vi "RTA4004_Oscilloscope_Fetch_2Ch_Waveform.vi"() -> ()   [LabVIEW 2017]
uses:
  <instrlib>/Rohde&Schwarz RTx Oscilloscopes/Rohde&Schwarz RTx Oscilloscopes.lvlib
panel:
  in  "Requested Record Length":i32=2000000
  out "Waveform CH2":T1(graph) caption="Waveform"
  in  "Record":bool
  in  "Description":string[](array[string])=["Measurement", "Near Football Field"]
  out "Record File Name":string
  in  "Channel 2":i32=2 caption="Channel (2)"
  out "Recorded Size":i32
  in  "Number of Loops":i32=1
  out "Current Loop":i32
  in  "Channel (1)":i32=1
  in  "Oscilloscope Resource Name":refnum<visa-resource-name>="TCPIP::192.168.10.205::INSTR" caption="VISA resource name"
  in  "Reset":bool
  in  "ID Query":bool=TRUE
  out "Waveform CH1":T1(graph) caption="Waveform"
  # "Rohde & Schwarz RTM2000 Oscilloscope Read Waveform Example"
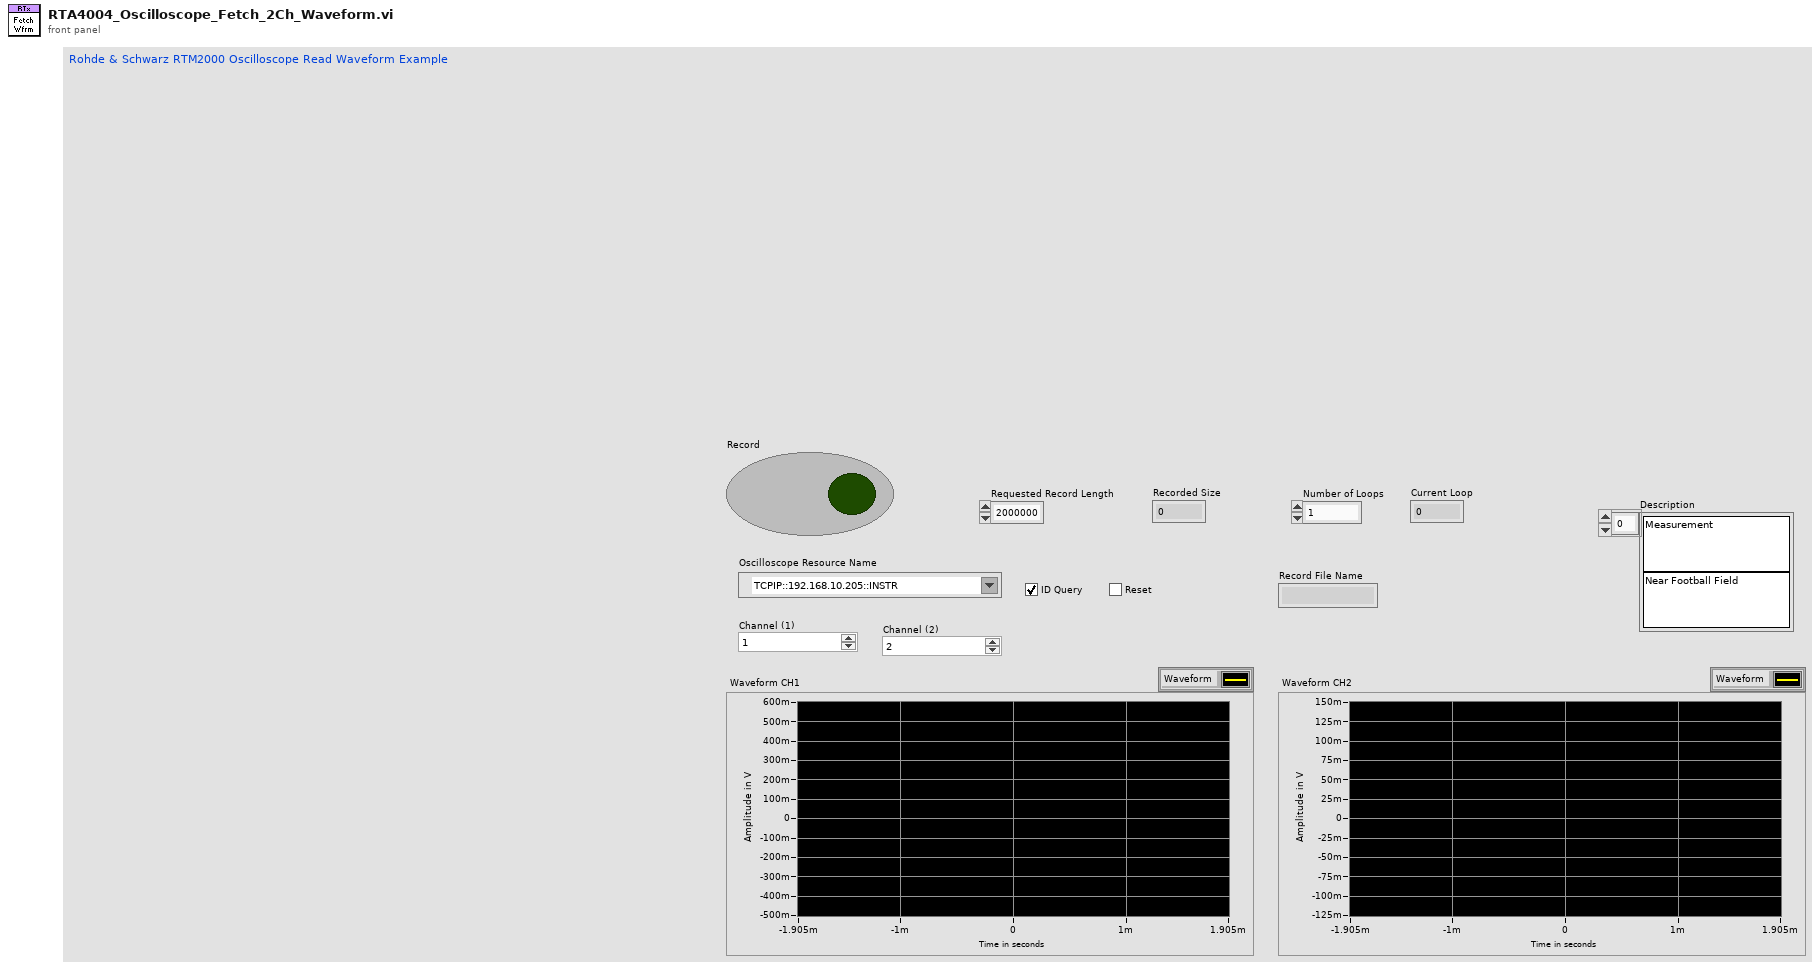
[diagram p1: front panel]
types:
  T1 = cluster{"Initial X":dbl, "X Increment":dbl, "Waveform Array":dbl[]}
  T2 = enum16{"open", "open or create", "create or replace", "create", "open (read-only)"}
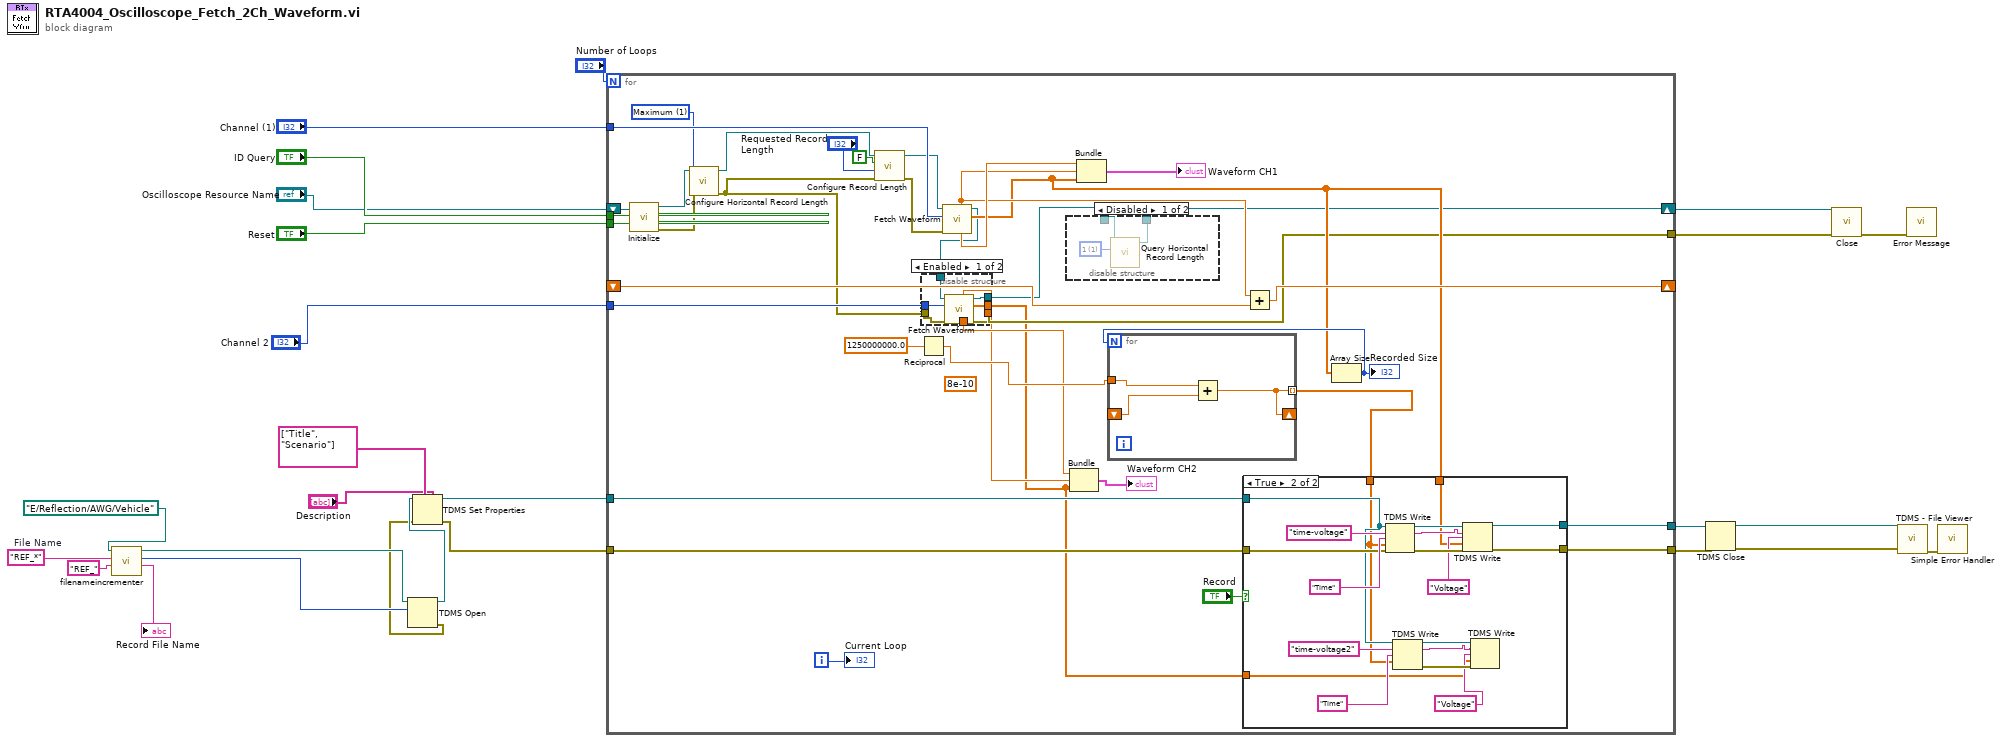
[diagram p0: block diagram]
diagram:
  w12 = "REF_*"  # File Name
  n1 = call "filenameincrementer.vi"("string"="REF_", "pattern"=w12, "Path"=path "E:/Reflection/AWG/Vehicle" ("file path")) -> ("File Name"=→"Record File Name":string, "Operation"=w8:T2, "File Path"=w7:path)  [unwired: 6 in]
  n2 = TDMS Open(10:w8, 11:w7) -> (0:w2:errorcluster, 3:w4:refnum<k34>)  [unwired: 5 in]
  n3 = TDMS Set Properties(5:"Description", 7:string[] ["Title", "Scenario"], 8:w2, 11:w4) -> (0:w1:errorcluster, 3:w3:refnum<k34>)  [unwired: 2 in, 2 out]
  n4 = for {
    N: "Number of Loops" -> [_]
    tunnel: "Reset" -> [w63]
    tunnel: "ID Query" -> [w62]
    tunnel: "Channel (1)" -> [w61]
    tunnel: [w47] -> w23
    shift-right: [w34] -> w17
    shift-left: "Oscilloscope Resource Name" -> [w58]
    tunnel: [w53] -> w15
    tunnel: [w52] -> w14
    shift-right: [w54] -> _
    shift-left: _ -> [w55]
    tunnel: "Channel 2" -> [w44]
    tunnel: w3 -> [w42]
    tunnel: w1 -> [w43]
    i -> [w59]
    w37 = 1 items=["Default", "Maximum", "Display Maximum"] ("Record Length (Default)")
    (unwired) 8e-10 ("x")
    n5 = call <instrlib>:"Initialize.vi"("Reset (T: Reset)"=w63, "ID Query (T: Check)"=w62, "VISA resource name"=w58) -> ("error out"=w30:errorcluster, "VISA resource name out"=w36:refnum<visa-resource-name>)  [unwired: 7 in]
    n6 = call <instrlib>:"Configure Horizontal Record Length.vi"("error in (no error)"=w30, "Record Length (Default)"=w37, "VISA resource name"=w36) -> ("error out"=w29:errorcluster, "VISA resource name out"=w33:refnum<visa-resource-name>)  [unwired: 7 in]
    n7 = call <instrlib>:"Configure Record Length.vi"("error in (no error)"=w29, "Record Length (10000)"="Requested Record Length", "Automatic (T: On)"=FALSE, "VISA resource name"=w33) -> ("error out"=w28:errorcluster, "VISA resource name out"=w35:refnum<visa-resource-name>)  [unwired: 6 in]
    n8 = Reciprocal(x=1250000000.0) -> (1/x=w49:dbl)
    n9 = call <instrlib>:"Fetch Waveform.vi"("error in (no error)"=w28, "Channel (1)"=w61, "VISA resource name"=w35) -> ("Waveform Array"=w50:dbl[], "VISA resource name out"=w27:refnum<visa-resource-name>, "Initial X"=w57:dbl, "X Increment"=w56:dbl)  [unwired: 4 in, 1 out]
    n10 = disable-structure shown="Enabled" {
      disable-tunnel: [w74 _] -> w47
      disable-tunnel: [w73 _] -> w46
      disable-tunnel: [w72 _] -> w45
      disable-tunnel: w44 -> [w71 _]
      disable-tunnel: [w70 _] -> w41
      disable-tunnel: [w69 _] -> w34
      disable-tunnel: w29 -> [w68 _]
      disable-tunnel: w27 -> [w67 _]
      frame Enabled {
        n11 = call <instrlib>:"Fetch Waveform.vi"("error in (no error)"=w68, "Channel (1)"=w71, "VISA resource name"=w67) -> ("error out"=w74:errorcluster, "Waveform Array"=w70:dbl[], "VISA resource name out"=w69:refnum<visa-resource-name>, "Initial X"=w73:dbl, "X Increment"=w72:dbl)  [unwired: 4 in]
      }
      frame Disabled {
      }
    }
    n12 = disable-structure shown="Disabled" {
      disable-tunnel: _ -> [w66 _]
      disable-tunnel: [w65 _] -> _
      frame Disabled {
        w64 = 1 items=["1"=1, "2"=2, "3"=3, "4"=4, "External"=5] ("Channel (1)")
        n13 = call <instrlib>:"Query Horizontal Record Length.vi"("Channel (1)"=w64, "VISA resource name"=w66) -> ("VISA resource name out"=w65:refnum<visa-resource-name>)  [unwired: 7 in, 2 out]
      }
      frame Enabled {
      }
    }
    n14 = Bundle("Initial X"=w46, "X Increment"=w45, "Waveform Array"=w41) -> (→"Waveform CH2":T1)  [unwired: 1 in]
    n15 = Bundle("Initial X"=w57, "X Increment"=w56, "Waveform Array"=w50) -> (→"Waveform CH1":T1)  [unwired: 1 in]
    n16 = Add(x=w56, y=w55) -> (x+y=w54:dbl)
    n17 = Array Size(array=w50) -> (size(s)=w51:i32)
    "Recorded Size" <- w51
    n18 = for {
      N: w51 -> [_]
      tunnel: w49 -> [w98]
      tunnel: [w97] -> w40 mode=indexing
      shift-right: [w97] -> _
      shift-left: _ -> [w96]
      n19 = Add(x=w98, y=w96) -> (x+y=w97:dbl)
    }
    n20 = case shown="True" "Record" {
      tunnel: [w76 w93] -> w53
      tunnel: [w75 w91] -> w52
      tunnel: w50 -> [_ w87]
      tunnel: w43 -> [w75 w86]
      tunnel: w42 -> [w76 w81]
      tunnel: w41 -> [_ w78]
      tunnel: w40 -> [_ w77]
      frame False {
      }
      frame True {
        n21 = TDMS Write(0:w81, 5:"time-voltage" ("group name in (Untitled)"), 7:"Time", 9:w77, 11:w86) -> (4:w94:refnum<k34>, 6:w88:string, 15:w92:errorcluster)  [unwired: 1 in, 1 out]
        n22 = TDMS Write(0:w81, 5:"time-voltage2" ("group name in (Untitled)"), 7:"Time", 9:w77) -> (4:w82:refnum<k34>, 6:w85:string, 15:w83:errorcluster)  [unwired: 2 in, 1 out]
        n23 = TDMS Write(0:w94, 5:w88, 7:"Voltage", 9:w87, 11:w92) -> (4:w93:refnum<k34>, 15:w91:errorcluster)  [unwired: 1 in, 2 out]
        n24 = TDMS Write(0:w82, 5:w85, 7:"Voltage", 9:w78, 11:w83) -> ()  [unwired: 1 in, 4 out]
      }
    }
    "Current Loop" <- w59
  }
  n25 = TDMS Close(8:w14, 11:w15) -> (0:w19:errorcluster, 3:w20:path)
  n26 = call <instrlib>:"Close.vi"("error in (no error)"=w23, "VISA resource name"=w17) -> ("error out"=w22:errorcluster)  [unwired: 9 in]
  n27 = call <vilib>:"TDMS - File Viewer.vi"("error in (no error)"=w19, "file path"=w20) -> ("error out"=w21:errorcluster)  [unwired: 4 in, 1 out]
  n28 = call <instrlib>:"Error Message.vi"("error in (no error)"=w22) -> ()  [unwired: 10 in, 5 out]
  n29 = call <vilib>:"Simple Error Handler.vi"("error in (no error)"=w21) -> ()  [unwired: 4 in, 5 out]
